vi "PS35_SimpleConnect.vi"(2 "error in (no error)":errorcluster, 3 "Serial number":string, 4 "Control unit ID":i32=1 min=1 max=20) -> (0 "error out":errorcluster)   [LabVIEW 2020]
doc: "PS35_SimpleConnect.vi, created: 03.03.2009 alex; last change: 22.10.2019 alex;\n\n<B>FUNCTION:</B> \n\nFind control unit with the specified serial number and connect to it.\n*Serial interface (communication via USB or serial port)*\nThe application software can access this interface in the same way as \nit would access a standard serial port (COM). The parameters for Baudrate, \nParity, Databits and Stopbits are predefined (9600, no parity, 8 databits, 1 stopbit).\nThe software handshake character is CR.\n*Ethernet interface (communication via Com-Server)*\nAs Com-Server the OWIS software tool \"OWISerialServer.exe\" may be used\n(..\\OWISoft\\Application\\system). The application software can access \nthis interface via Windows TCP socket: special communication for OWIS software\n(command + delay). The software handshake character is CR.\n----------------------------------------------------------------------------------------\n<B>INPUT:</B>\n[I32] <B>Control unit ID:</B> control unit index 1-10. (Default=1, Range=1...20) \n11...20 - debug mode\n1...10 - standard mode\n[CStr] <B>Serial number:</B> control unit serial number. (Default=empty string)\nUSB or serial port\nempty string - the first found control unit is connected;\n\"12345678\" - control unit with the specified serial number is connected;\nEthernet interface\n\"net\" - control unit is connected to the Com-Server (local application) \nby the first found local IP address and port number 1200.\n[CLU] <B>error in</B>\n----------------------------------------------------------------------------------------\n<B>OUTPUT:</B>\n[CLU] <B>error out</B>\n0 - no error,\n1 - function error (invalid parameters),\n5 - no response from control unit (check cable, connection or reset control unit),\n7 - control unit with the specified serial number is not found,\n9 - no connection to tcp/ip socket.\n----------------------------------------------------------------------------------------\n<B>SUB-VIs:</B>\n----------------------------------------------------------------------------------------\n<B>EXT-Calls:</B>\nps35.dll (V2.01)\n----------------------------------------------------------------------------------------"
uses:
  ps35.dll
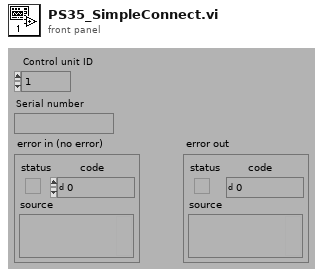
[diagram p1: front panel]
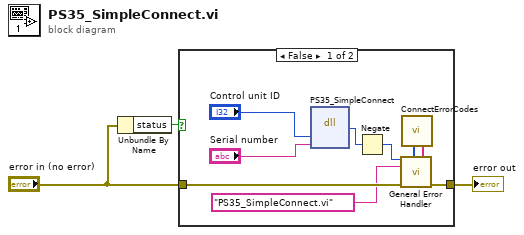
[diagram p0: block diagram]
diagram:
  n1 = Unbundle By Name("error in (no error)") -> ("status"=w1:bool)
  n2 = case shown="False" w1 {
    tunnel: "error in (no error)" -> [w11 w13]
    tunnel: [w10 w13] -> w3
    frame False {
      n3 = dll-call lib="C:/GEECS/Developers Version/source/Device Drivers/OwiSoft/OWISoftOEM/ps35/labview/lv82/ps35.dll" fn="PS35_SimpleConnect"("Index"="Control unit ID", "szSerNum"="Serial number") -> ("Rückgabetyp"=w9:i32)  [unwired: 5 in, 2 out]
      n4 = Negate(x=w9) -> (-x=w6:i32)
      n5 = call "ConnectErrorCodes.vi"() -> ("[user-defined codes]"=w5:i32[], "[user-defined descriptions]"=w4:string[])  [unwired: 8 in]
      n6 = call <vilib>:"General Error Handler.vi"("[error code] (0)"=w6, "[user-defined codes]"=w5, "[user-defined descriptions]"=w4, "[error source] (\" \")"="PS35_SimpleConnect.vi", "error in (no error)"=w11) -> ("error out"=w10:errorcluster)  [unwired: 6 in, 4 out]
    }
    frame True {
    }
  }
  "error out" <- w3
